vi "DB-文件创建.vi"(8 "错误常量":errorcluster, 11 "文件路径输入控件":path) -> (0 "错误输出":errorcluster, 2 "已存在？":bool caption="文件存在？", 3 "DB路径 o":path=path "D:/MyAccessDB.mdb" caption="ACCESS数据库MDB文件")   [LabVIEW 2017]
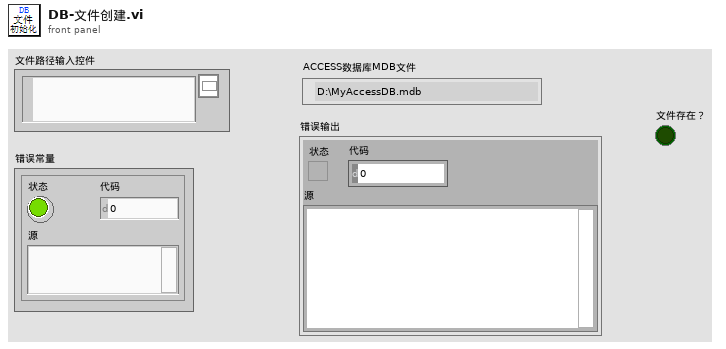
[diagram p1: front panel]
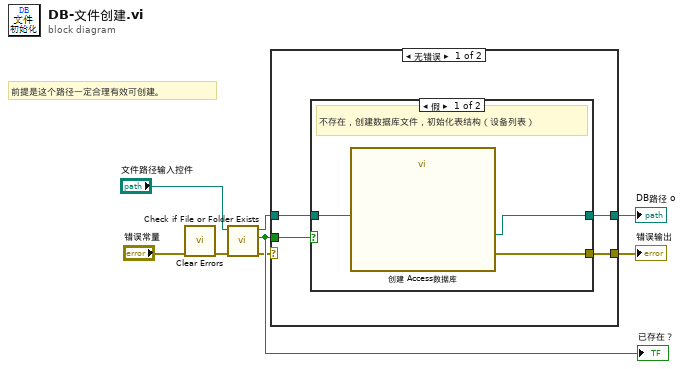
[diagram p0: block diagram]
diagram:
  # "前提是这个路径一定合理有效可创建。"
  n1 = call <vilib>:"Clear Errors.vi"("error in (no error)"="错误常量") -> ("error out"=w1:errorcluster)  [unwired: 5 in, 1 out]
  n2 = call <vilib>:"Check if File or Folder Exists.vi"("error in (no error)"=w1, "path"="文件路径输入控件") -> ("error out"=w5:errorcluster, "file or folder exists?"=w7:bool, "dup path"=w6:path)  [unwired: 7 in]
  "已存在？" <- w7
  n3 = case shown="无错误" w5 {
    selector: w5 -> [_ w18]
    tunnel: w7 -> [w12 _]
    tunnel: w6 -> [w11 w17]
    tunnel: [w10 w17] -> w4
    tunnel: [w9 w18] -> w3
    frame No Error {
      n4 = case shown="假" w12 {
        tunnel: [w14 w16] -> w10
        tunnel: w11 -> [w15 w16]
        tunnel: [w13 _] -> w9
        frame False {
          # "不存在，创建数据库文件，初始化表结构（设备列表）"
          n5 = call "创建 Access数据库.vi"("路径 i"=w15) -> ("错误输出"=w13:errorcluster, "路径 o"=w14:path)  [unwired: 9 in]
        }
        frame True {
          # "存在，路径传递"
        }
      }
    }
    frame Error {
    }
  }
  "DB路径 o" <- w4
  "错误输出" <- w3
